vi "DriveEnable.vi"(0 "Axis In (Axis Space)":T1=enum."Axis Space", 5 "Enable (T)":bool=TRUE, 11 "error in (no error)":errorcluster) -> (4 "Axis Out":T1, 15 "error out":errorcluster)   [LabVIEW 2009]
uses:
  typedefs/AxisSelect_Enum.ctl
  typedefs/Ultra3000/Cmds.ctl
  typedefs/Ultra3000/Func.ctl
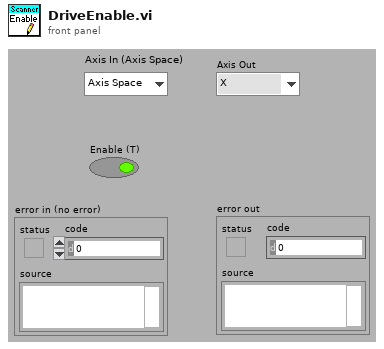
[diagram p1: front panel]
types:
  T1 = typedef "AxisSelect_Enum.ctl" = enum16{"X", "Y", "Z", "Axis Space"}
  T2 = typedef "Func.ctl" = u16
  T3 = typedef "Cmds.ctl" = u16
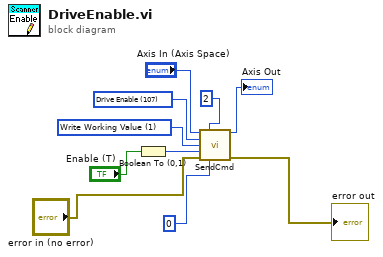
[diagram p0: block diagram]
diagram:
  w9 = T2 1 items=["Read Working Value", "Write Working Value", "Read Non-Volatile Value", "Write Non-Volatile and Woring Value", "Copy Non-Volatile Value to Working Value", "Copy Working Value to Non-Volatile Value", "Read Default Value", "Copy Default Value to Non-Volatile and Working Values", "Read Min Value", "Read Max Value", "Read Array Index Min", "Read Array Index Max"] ("Function")
  w5 = T3 107 items=["Power-Up Status"=1, "Drive Name"=6, "Position Window Size"=22, "Position Window Time"=23, "Zero SPeed Limit"=34, "Speed Window Size"=35, "Up to Speed Limit"=37, "Forward Current Limit"=47, "Reverse Current Limit"=48, "Override Mode"=67, "Operation Mode"=90, "Host Control Mode"=97, "Reset Drive"=106, "Drive Enable"=107, "Setpoint Current"=108, "Setpoint Velocity"=109, "Setpoint Acceleration"=110, "Reset Faults"=111, "Position Comparator"=349, "Postition Comparator Polarity"=350, "Position Rollover Enable"=404, "Baud Rate"=80, "Frame Format"=81, "Drive Address"=82, "Broadcast Address"=83, "Auto-start Indexing"=88, "Start Index"=112, "Host Index"=184, "Index Type"=174, "Index Dist/Pos"=175, "Index Reg Dist"=176, "Index Velocity"=177, "Index Acceleration"=178, "Index Deceleration"=179, "Index Dwell"=180, "Index Count"=181, "Index Termination"=182, "Index Pointer"=183, "Index Abort Deceleration"=185, "Positive Soft Pos Limit"=216, "Negative Soft Pos Limit"=217] ("Command")
  n1 = Boolean To (0,1)(Boolean="Enable (T)") -> (0, 1=w7:i16)
  n2 = call "SendCmd.vi"("Axis In"="Axis In (Axis Space)", "Data Length Constant (0)"=u8 2 ("DLC"), "Command"=w5, "Function"=w9, "Data (0)"=w7, "error in (no error)"="error in (no error)", "Index (0)"=u8 0 ("Index")) -> ("Axis Out"=→"Axis Out":T1, "error out"=→"error out":errorcluster)  [unwired: 5 in, 2 out]
